vi "Set Servos.vi"(0 "comm interface in":refnum<class "Pixy Com.lvclass">, 5 "servo 0 (pan)":u16 max=511, 7 "servo 1 (tilt)":u16 max=511, 11 "error in":errorcluster) -> (4 "comm interface out":refnum<class "Pixy Com.lvclass">, 15 "error out":errorcluster)   [LabVIEW 2018, in "Pixy2.lvlib"]
doc: "Sets the servo value for the pan and tilt servos."
uses:
  Pixy2.lvlib
  Interface/Pixy Com.lvclass
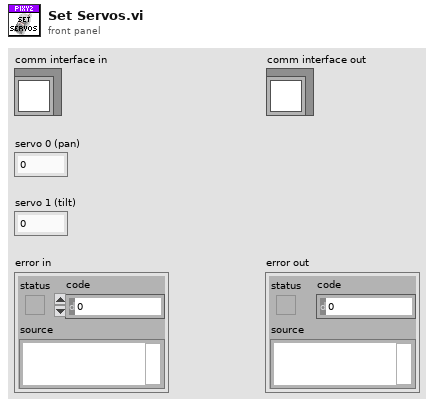
[diagram p1: front panel]
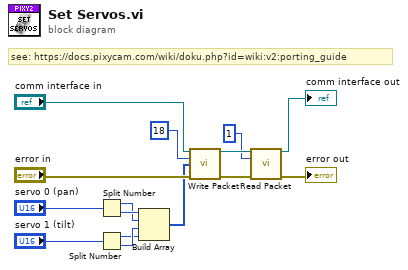
[diagram p0: block diagram]
diagram:
  # "see: https://docs.pixycam.com/wiki/doku.php?id=wiki:v2:porting_guide"
  n1 = Split Number(x="servo 0 (pan)") -> (hi(x)=w4:u8, lo(x)=w5:u8)
  n2 = Split Number(x="servo 1 (tilt)") -> (hi(x)=w2:u8, lo(x)=w3:u8)
  n3 = Build Array(w5, w4, w3, w2) -> (w1:u8[])
  n4 = call "Write Packet.vi"("comm interface in"="comm interface in", "type"=u8 18, "payload"=w1, "error in"="error in") -> ("comm interface out"=w12:refnum<class "Pixy Com.lvclass">, "error out"=w13:errorcluster)  [unwired: 10 in]
  n5 = call "Read Packet.vi"("comm interface in"=w12, "expected type"=u8 1, "error in"=w13) -> ("comm interface out"=→"comm interface out":refnum<class "Pixy Com.lvclass">, "error out"=→"error out":errorcluster)  [unwired: 9 in, 2 out]
